vi "GUNSC_responseToQ.vi"(8 "error in":errorcluster, 11 "queue name":string) -> (0 "error out":errorcluster)   [LabVIEW 2014]
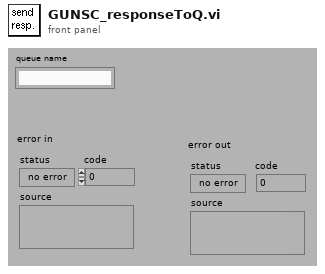
[diagram p1: front panel]
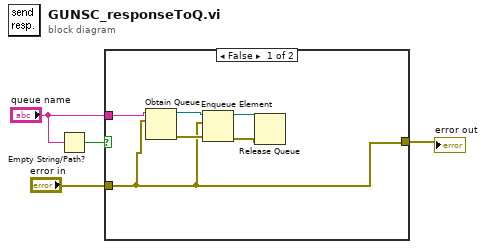
[diagram p0: block diagram]
diagram:
  n1 = Empty String/Path?(string/path="queue name") -> (empty?=w3:bool)
  n2 = case shown="False" w3 {
    tunnel: "queue name" -> [w10 _]
    tunnel: "error in" -> [w5 w11]
    tunnel: [w5 w11] -> w1
    frame False {
      n3 = Obtain Queue(name (unnamed)=w10, element data type=w5) -> (queue out=w9:refnum<queue>, error out=w8:errorcluster)  [unwired: 3 in, 1 out]
      n4 = Enqueue Element(queue=w9, element=w5, error in (no error)=w8) -> (queue out=w7:refnum<queue>, error out=w6:errorcluster)  [unwired: 2 out]
      n5 = Release Queue(queue=w7, error in (no error)=w6) -> ()  [unwired: 4 out]
    }
    frame True {
    }
  }
  "error out" <- w1
